vi "TimeKeeper(ms).vi"(7 "Reset?(F)":bool, 8 "error in (no error)":errorcluster, 11 "Period(ms)":i32=50) -> (0 "error out":errorcluster, 1 "Idle(ms)":i32, 2 "Used(ms)":i32)   [LabVIEW 2017]
doc: "Holds for the configured period while returning the elapsed time, so a loop can be paced to a fixed period. Wire Reset?(F) to restart."
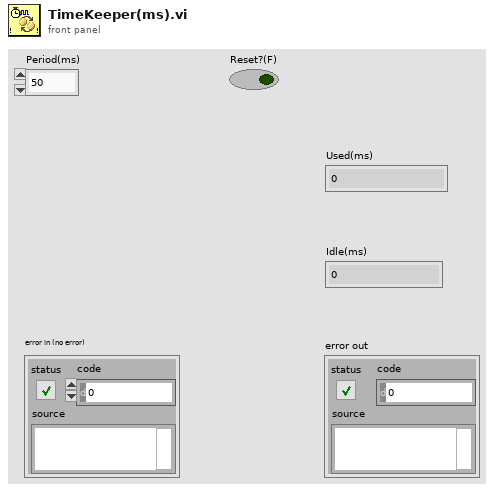
[diagram p1: front panel]
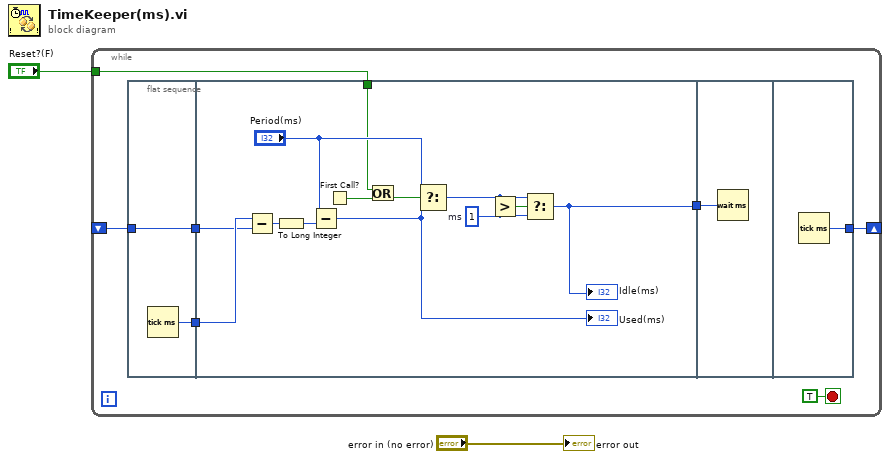
[diagram p0: block diagram]
diagram:
  n1 = while {
    shift-right: [w5] -> _
    shift-left: _ -> [w6]
    tunnel: "Reset?(F)" -> [w3]
    stop <- TRUE stop-if-true
    n2 = flat-sequence {
      tunnel: [w11] -> w8
      tunnel: [w10] -> w7
      tunnel: w6 -> [w10]
      tunnel: w8 -> [w16]
      tunnel: w7 -> [w15]
      tunnel: [w14] -> w4
      tunnel: w3 -> [w12]
      tunnel: w4 -> [w25]
      tunnel: [w26] -> w5
      frame #0 {
        n3 = Tick Count (ms)() -> (millisecond timer value=w11:u32)
      }
      frame #1 {
        w17 = 1  # ms
        n4 = Subtract(x=w16, y=w15) -> (x-y=w19:u32)
        n5 = To Long Integer(number=w19) -> (32bit integer=w18:i32)
        n6 = Subtract(x="Period(ms)", y=w18) -> (x-y=w21:i32)
        "Used(ms)" <- w21
        n7 = First Call?() -> (First Call?: T/F=w20:bool)
        n8 = Or(x=w12, y=w20) -> (x .or. y?=w13:bool)
        n9 = Select(t="Period(ms)", s=w13, f=w21) -> (s? t:f=w23:i32)
        n10 = Greater?(x=w23, y=w17) -> (0:w22:bool)
        n11 = Select(t=w23, s=w22, f=w17) -> (s? t:f=w14:i32)
        "Idle(ms)" <- w14
      }
      frame #2 {
        n12 = Wait (ms)(milliseconds to wait=w25) -> ()  [unwired: 1 out]
      }
      frame #3 {
        n13 = Tick Count (ms)() -> (millisecond timer value=w26:u32)
      }
    }
  }
  "error out" <- "error in (no error)"
